vi "SVM_Sweep.vi"(0 "Data IN":dbl[](graph), 5 "time step":dbl, 7 "Angle (degrees)":dbl=90.0, 9 "SVs":i32) -> (2 "PTs":i32[](array[numeric]), 3 "SVM Out Stack":T1(array[cluster]), 4 "SVM Fit Stack":T2(array[cluster]), 6 "SV Gaps":cluster{i32, "x":i32, dbl[][]}, 8 "Max Index":i32[](array[numeric]), 10 "SVM Size (um)":cluster{i32, "x":i32, dbl[][]}, 14 "Array":cluster{"A tau":dbl[]}[](array[cluster]), 15 "Best Size":i32[](array[numeric]))   [LabVIEW 2022 SP3]
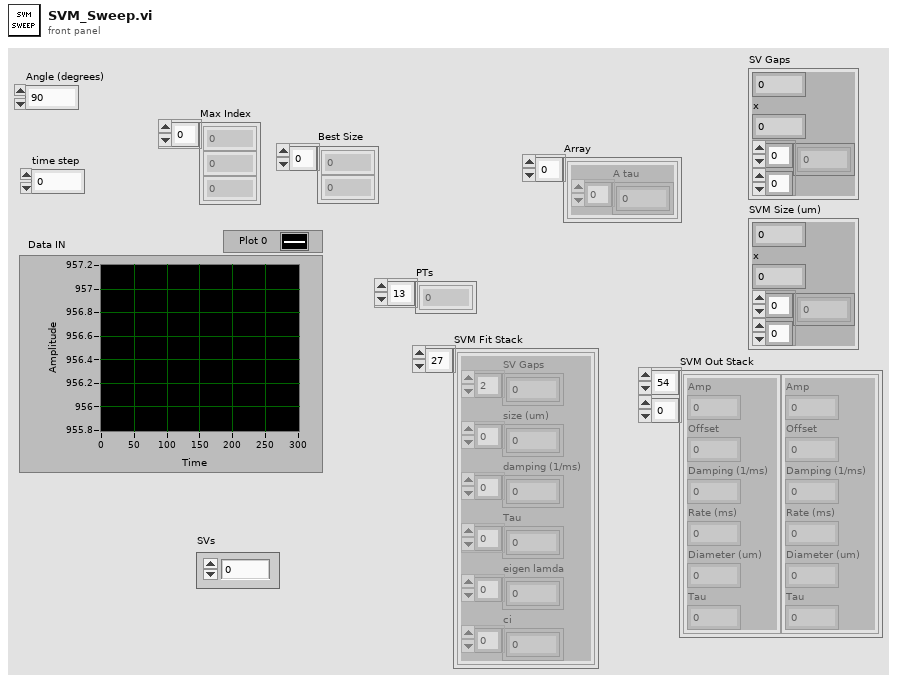
[diagram p1: front panel]
types:
  T1 = cluster{"Amp":dbl, "Offset":dbl, "Damping (1/ms)":dbl, "Rate (ms)":dbl, "Diameter (um)":dbl, "Tau":dbl}[][]
  T2 = cluster{"SV Gaps":dbl[], "size (um)":dbl[], "damping (1/ms)":dbl[], "Tau ":cdb[], "eigen lamda":dbl[], "ci":dbl[]}[]
  T3 = cluster{"SV Gaps":dbl[], "size (um)":dbl[], "damping (1/ms)":dbl[], "Tau ":cdb[], "eigen lamda":dbl[], "ci":dbl[]}
  T4 = cluster{"Amp":dbl, "Offset":dbl, "Damping (1/ms)":dbl, "Rate (ms)":dbl, "Diameter (um)":dbl, "Tau":dbl}[]
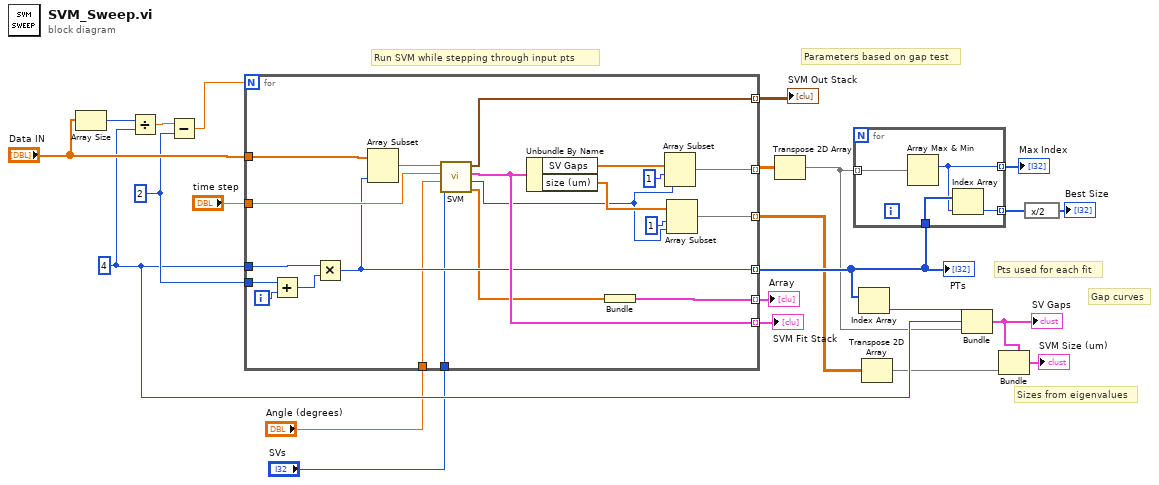
[diagram p0: block diagram]
diagram:
  w15 = 2 ("x")
  w9 = 4 ("x")
  # "Pts used for each fit"
  # "Sizes from eigenvalues"
  # "Gap curves"
  # "Parameters based on gap test"
  # "Run SVM while stepping through input pts"
  n1 = Array Size(array="Data IN") -> (size(s)=w18:i32)
  n2 = Divide(x=w18, y=w9) -> (x/y=w17:dbl)
  n3 = Subtract(x=w17, y=w15) -> (x-y=w16:dbl)
  n4 = for {
    N: w16 -> [_]
    tunnel: "Data IN" -> [w42]
    tunnel: "time step" -> [w40]
    tunnel: [w35] -> w8 mode=indexing
    tunnel: [w34] -> w6 mode=indexing
    tunnel: [w33] -> w21 mode=indexing
    tunnel: [w32] -> w22 mode=indexing
    tunnel: [w27] -> w14 mode=indexing
    tunnel: [w31] -> w11 mode=indexing
    tunnel: w9 -> [w30]
    tunnel: w15 -> [w29]
    tunnel: "Angle (degrees)" -> [w25]
    tunnel: "SVs" -> [w24]
    i -> [w44]
    n5 = Add(x=w29, y=w44) -> (x+y=w43:i32)
    n6 = Multiply(x=w30, y=w43) -> (x*y=w31:i32)
    n7 = Array Subset(array=w42, length=w31) -> (w41:dbl[])  [unwired: 1 in]
    n8 = call "SVM.vi"("SVs"=w24, "Angle (degrees)"=w25, "time step"=w40, "Data IN"=w41) -> ("A tau"=w28:dbl[], "GapCutOff"=w26:i16, "SVM Out"=w32:T3, "Array"=w33:T4)  [unwired: 4 in]
    n9 = Unbundle By Name(w32) -> ("SV Gaps"=w38:dbl[], "size (um)"=w36:dbl[])
    n10 = Bundle("A tau"=w28) -> (w27:cluster{"A tau":dbl[]})  [unwired: 1 in]
    n11 = Array Subset(array=w38, index=1, length=w26) -> (w35:dbl[])
    n12 = Array Subset(array=w36, index=1, length=w26) -> (w34:dbl[])
  }
  "SVM Fit Stack" <- w22
  "SVM Out Stack" <- w21
  "PTs" <- w11
  "Array" <- w14
  n13 = Transpose 2D Array(2D array=w8) -> (transposed array=w3:dbl[][])
  n14 = for {
    tunnel: w3 -> [w48] mode=indexing
    tunnel: [w45] -> w20 mode=indexing
    tunnel: w11 -> [w47]
    tunnel: [w46] -> w12 mode=indexing
    n15 = Array Max & Min(array=w48) -> (max index (indices)=w45:i32)  [unwired: 3 out]
    n16 = Index Array(array=w47, index=w45) -> (element=w46:i32)
  }
  "Max Index" <- w20
  n17 = Index Array(array=w11) -> (element=w10:i32)  [unwired: 1 in]
  n18 = Transpose 2D Array(2D array=w6) -> (transposed array=w4:dbl[][])
  n19 = Bundle(w10, "x"=w9, w3) -> (w7:cluster{i32, "x":i32, dbl[][]})  [unwired: 1 in]
  "SV Gaps" <- w7
  n20 = Bundle(cluster=w7, w4) -> (→"SVM Size (um)":cluster{i32, "x":i32, dbl[][]})  [unwired: 2 in]
  n21 = expression code="x/2"(w12) -> (→"Best Size":i32[])
